vi "Read Device.vi"(8 "error in (no error)":errorcluster) -> (0 "error out":errorcluster, 2 "Humidity (unit?)":dbl, 3 "Temperature (unit?)":dbl)   [LabVIEW 2016, in "TEMPerHUM.lvlib"]
uses:
  TEMPerHUM.lvlib
  RDingUSB.dll
panel:
  out "Read work?":bool
  out "Write work?":bool
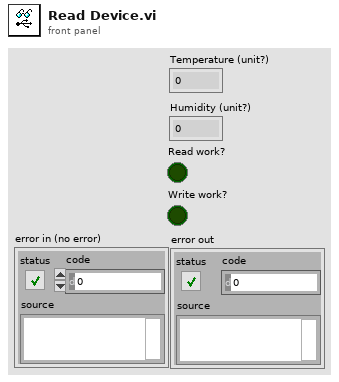
[diagram p1: front panel]
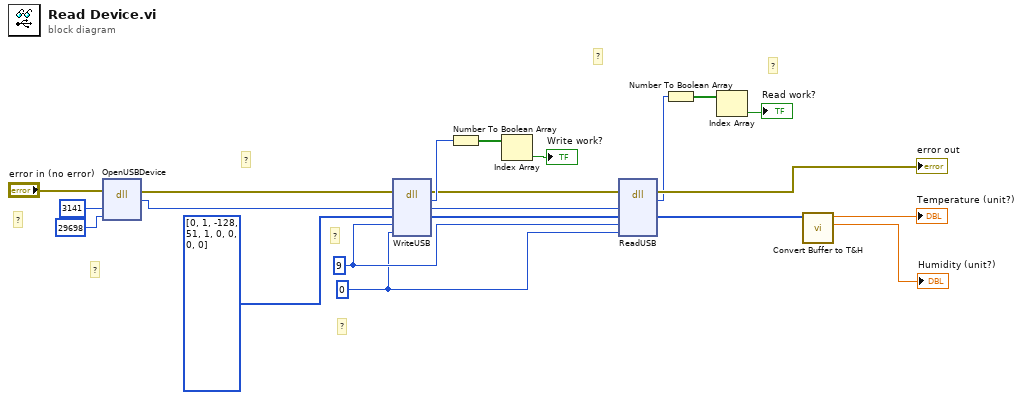
[diagram p0: block diagram]
diagram:
  w6 = u64 0 ("number0fBytesWrite")
  w8 = 9 ("bytesCount")
  # "?"
  # "?"
  # "?"
  # "?"
  # "?"
  # "?"
  # "?"
  n1 = dll-call lib="C:/Users/patrick/Documents/GitHub/TEMPerHUM/TEMPerHUM via DLL/TEMPerHUM/RDingUSB.dll" fn="OpenUSBDevice"(error in="error in (no error)", "VID"=3141, "PID"=29698) -> (error out=w19:errorcluster, "return type"=w20:i64)  [unwired: 4 in, 1 out]
  n2 = dll-call lib="C:/Users/patrick/Documents/GitHub/TEMPerHUM/TEMPerHUM via DLL/TEMPerHUM/RDingUSB.dll" fn="WriteUSB"(error in=w19, "deviceHandle"=w20, "buffer"=i8[] [0, 1, -128, 51, 1, 0, 0, 0, 0] ("Array"), "bytesCount"=w8, "number0fBytesWrite"=w6) -> (error out=w4:errorcluster, "return type"=w11:i32, "deviceHandle"=w9:i64, "buffer"=w7:i8[])  [unwired: 4 in, 1 out]
  n3 = Number To Boolean Array(number=w11) -> (Boolean array=w12:bool[])
  n4 = Index Array(array=w12) -> (element=→"Write work?":bool)  [unwired: 1 in]
  n5 = dll-call lib="C:/Users/patrick/Documents/GitHub/TEMPerHUM/TEMPerHUM via DLL/TEMPerHUM/RDingUSB.dll" fn="ReadUSB"(error in=w4, "deviceHandle"=w9, "buffer"=w7, "bytesCount"=w8, "number0fBytesRead"=w6) -> (error out=→"error out":errorcluster, "return type"=w16:i32, "buffer"=w17:u8[])  [unwired: 5 in, 1 out]
  n6 = Number To Boolean Array(number=w16) -> (Boolean array=w15:bool[])
  n7 = Index Array(array=w15) -> (element=→"Read work?":bool)  [unwired: 1 in]
  n8 = call "Convert Buffer to T&H.vi"("buffer"=w17) -> ("Humidity"=→"Humidity (unit?)":dbl, "Temperature"=→"Temperature (unit?)":dbl)  [unwired: 9 in]
